vi "note on.vi"() -> ()   [LabVIEW 2020]
uses:
  shared/midi note name.ctl
  366655e7-240c-4da6-9906-7197f63bd74a.vi
  midi out/midi out.lvclass
  shared/midi shared.lvlib
panel:
  out "MIDI Name":string
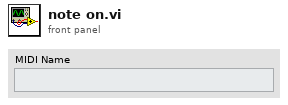
[diagram p1: front panel]
types:
  T1 = typedef "midi shared.lvlib/midi note name.ctl" = enum8{"C-1", "C#-1", "D-1", "D#-1", "E-1", "F-1", "F#-1", "G-1", "G#-1", "A-1", "A#-1", "B-1", "C0", "C#0", "D0", "D#0", "E0", "F0", "F#0", "G0", "G#0", "A0", "A#0", "B0", "C1", "C#1", "D1", "D#1", "E1", "F1", "F#1", "G1", "G#1", "A1", "A#1", "B1", "C2", "C#2", "D2", "D#2", "E2", "F2", "F#2", "G2", "G#2", "A2", "A#2", "B2", "C3", "C#3", "D3", "D#3", "E3", "F3", "F#3", "G3", "G#3", "A3", "A#3", "B3", "C4", "C#4", "D4", "D#4", "E4", "F4", "F#4", "G4", "G#4", "A4", "A#4", "B4", "C5", "C#5", "D5", "D#5", "E5", "F5", "F#5", "G5", "G#5", "A5", "A#5", "B5", "C6", "C#6", "D6", "D#6", "E6", "F6", "F#6", "G6", "G#6", "A6", "A#6", "B6", "C7", "C#7", "D7", "D#7", "E7", "F7", "F#7", "G7", "G#7", "A7", "A#7", "B7", "C8", "C#8", "D8", "D#8", "E8", "F8", "F#8", "G8", "G#8", "A8", "A#8", "B8", "C9", "C#9", "D9", "D#9", "E9", "F9", "F#9", "G9", "G#9", "A9", "A#9", "B9", "C10", "C#10", "D10", "D#10", "E10", "F10", "F#10", "G10"}
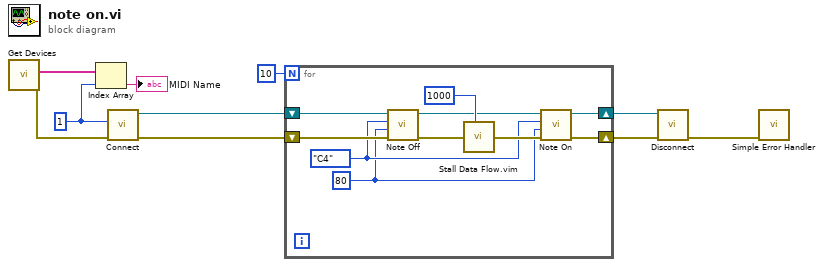
[diagram p0: block diagram]
diagram:
  w6 = 1 ("Device ID")
  n1 = call "Get Devices.vi"() -> ("error out"=w10:errorcluster, "Device Names"=w7:string[])  [unwired: 10 in]
  n2 = Index Array(array=w7, index=w6) -> (element=→"MIDI Name":string)
  n3 = call "Connect.vi"("error in (no error)"=w10, "Device ID"=w6) -> ("error out"=w8:errorcluster, "midi out out"=w9:refnum<class "midi out.lvclass">)  [unwired: 8 in]
  n4 = for {
    N: 10 -> [_]
    shift-right: [w14] -> w3
    shift-left: w9 -> [w20]
    shift-right: [w11] -> w2
    shift-left: w8 -> [w19]
    w12 = u8 80 ("Velocity (0-127)")
    w13 = midi_note_name."C4" ("MIDI Note Name")
    n5 = call "Note Off.vi"("error in (no error)"=w19, "Velocity (0-127)"=w12, "MIDI Note Name"=w13, "midi out in"=w20) -> ("error out"=w18:errorcluster, "midi out out"=w16:refnum<class "midi out.lvclass">)  [unwired: 6 in]
    n6 = call "Stall Data Flow.vim"("value in"=w18, "milliseconds to wait"=u32 1000) -> ("value out"=w15:errorcluster)  [unwired: 1 out]
    n7 = call "Note On.vi"("error in (no error)"=w15, "Velocity (0-127)"=w12, "MIDI Note Name"=w13, "midi out in"=w16) -> ("error out"=w11:errorcluster, "midi out out"=w14:refnum<class "midi out.lvclass">)  [unwired: 6 in]
  }
  n8 = call "Disconnect.vi"("error in (no error)"=w2, "midi out"=w3) -> ("error out"=w4:errorcluster)  [unwired: 9 in]
  n9 = call <vilib>:"Simple Error Handler.vi"("error in (no error)"=w4) -> ()  [unwired: 4 in, 5 out]
